vi "Create_Dataset(In3d_Out3D).vi"(4 "Read GTs?":bool, 5 "Input3D_Custom_Dims":T1, 6 "PreProcessing_Options":T2={"Image Type"=4, "Normalization Type"=enum."Standardize(DS_Stats)", "Interpolation Type"=1} {"Interpolation Type" items=["Zero Order", "Bi-Linear", "Quadratic", "Cubic Spline"]; "Image Type" items=["Grayscale (U8)", "Grayscale (I16)", "Grayscale (SGL)", "Complex (CSG)", "RGB (U32)", "HSL (U32)", "RGB (U64)", "Grayscale (U16)"]}, 7 "Dataset_Stats":T5 {"vars"."R" format="%#_3g"; "vars"."G" format="%#_3g"; "vars"."B" format="%#_3g"; "means"."R" format="%#_3g"; "means"."G" format="%#_3g"; "means"."B" format="%#_3g"}, 8 "error in (no error)":errorcluster, 9 "Good Unique Labels":string[](array[string]), 10 "GT Folder Path":path, 11 "Image File Paths":path[](array[path])) -> (0 "error out":errorcluster, 3 "Dataset(In3D_Out3D)":T7)   [LabVIEW 2020]
uses:
  <vilib>/Ngene/Deep Learning Toolkit/Toolkit/NN_Data/API/DataSet/DataSet_Types/NN_DataSet(In3D_Out3D).ctl
  <vilib>/Ngene/Deep Learning Toolkit/Toolkit/NN_Data/API/NN_Dims(C,H,W).ctl
  <vilib>/Ngene/Deep Learning Toolkit/Toolkit/NN_Data/Controls/DataRef_Types/4D/NN_Data_ref(4D_SGL).ctl
  PatchCore_AddOn/API/Controls/NNPC_DS_Stats.ctl
  PatchCore_AddOn/API/Controls/Image_Stats_RGB.ctl
  Controls/ImRead_PreProcessing_Options.ctl
  PatchCore_AddOn/Low_Level/Controls/Normalization_Type.ctl
  <vilib>/Ngene/Deep Learning Toolkit/Toolkit/Deep_Learning_Toolkit_by_Ngene.lvlib
  <vilib>/vision/NI_Vision_Development_Module.lvlib
  PatchCore_AddOn/PatchCore_AddOn.lvlib
panel:
  out "Imgs with missing GT":path[](array[path])
  out "Progress":i32
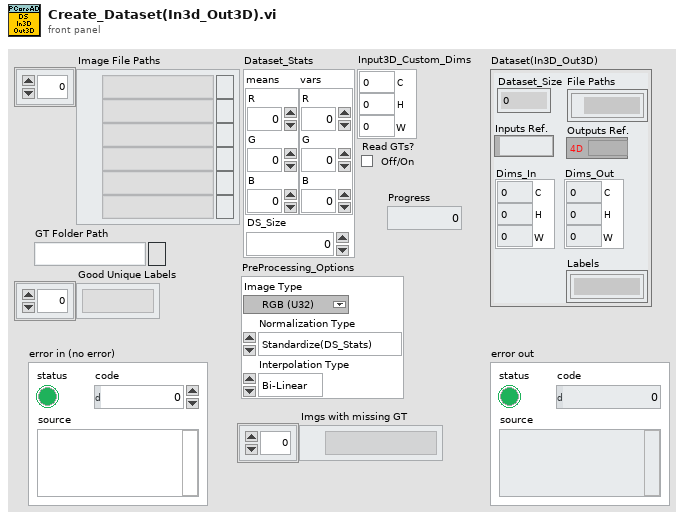
[diagram p1: front panel]
types:
  T1 = typedef "Deep_Learning_Toolkit_by_Ngene.lvlib/NN_Dims(C,H,W).ctl" = cluster{"C":i32, "H":i32, "W":i32}
  T2 = typedef "ImRead_PreProcessing_Options.ctl" = cluster{"Image Type":T3, "Normalization Type":T4, "Interpolation Type":u32}
  T3 = typedef "Image Type" = u32
  T4 = typedef "PatchCore_AddOn.lvlib/Normalization_Type.ctl" = enum16{"Standardize(DS_Stats)", "Standardize(Image_Stats)"}
  T5 = typedef "PatchCore_AddOn.lvlib/NNPC_DS_Stats.ctl" = cluster{"means":T6, "vars":T6, "DS_Size":i32}
  T6 = typedef "PatchCore_AddOn.lvlib/Image_Stats_RGB.ctl" = cluster{"R":sgl, "G":sgl, "B":sgl}
  T7 = typedef "Deep_Learning_Toolkit_by_Ngene.lvlib/NN_DataSet(In3D_Out3D).ctl" = cluster{"Dataset_Size":i32, "Dims_In":T1, "Labels":string[], "File Paths":path[], "Outputs Ref.":T8, "Inputs Ref.":variant, "Dims_Out":T1}
  T8 = typedef "Deep_Learning_Toolkit_by_Ngene.lvlib/NN_Data_ref(4D_SGL).ctl" = refnum<data-value>
  T9 = typedef "IMAQ Image.ctl" = refnum<image>
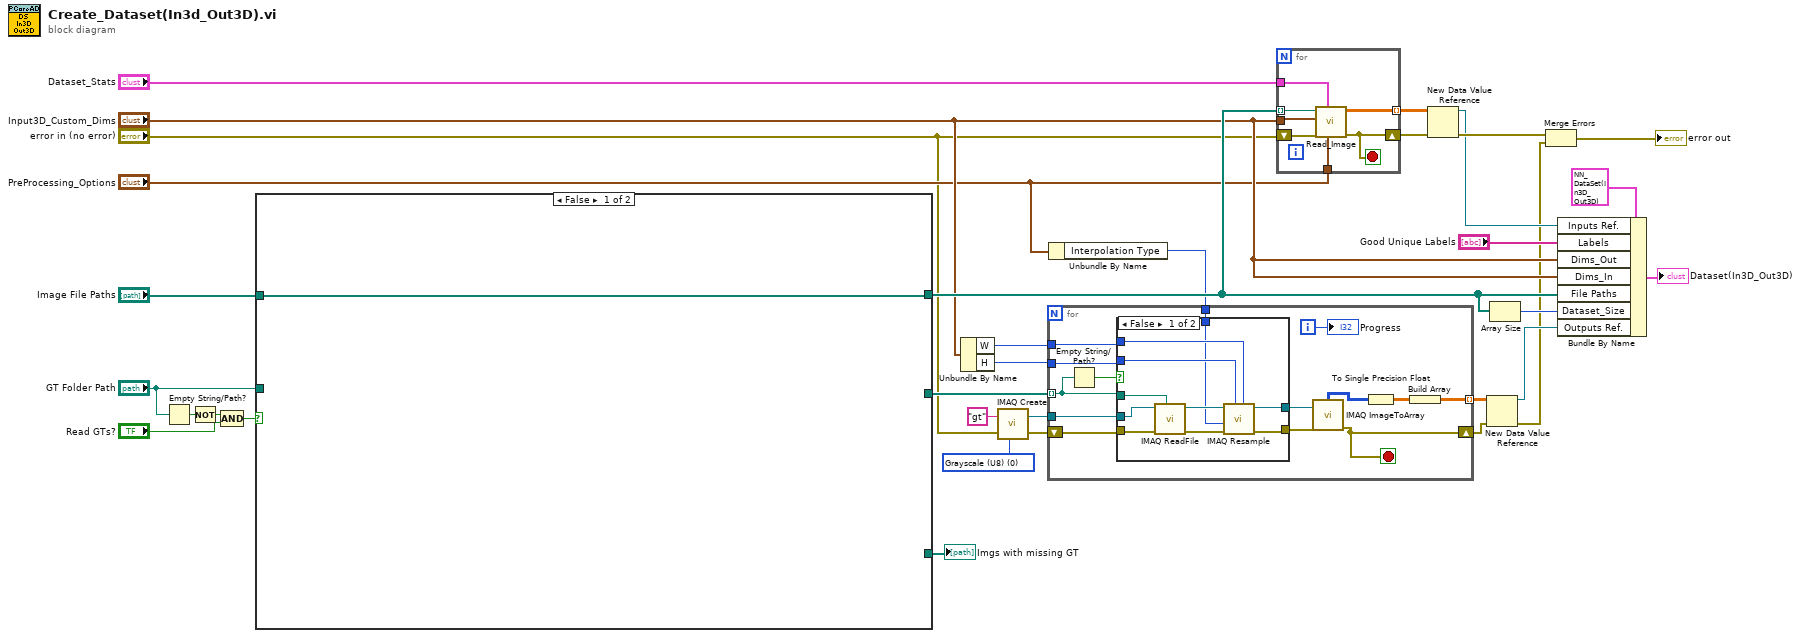
[diagram p0: block diagram]
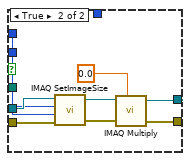
[diagram p2: hidden frame]
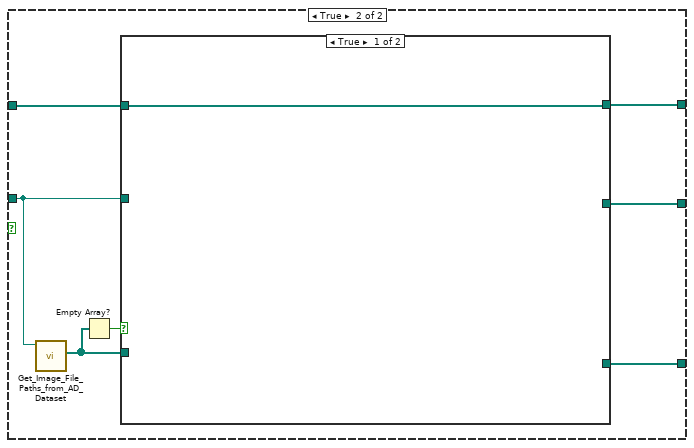
[diagram p3: hidden frame]
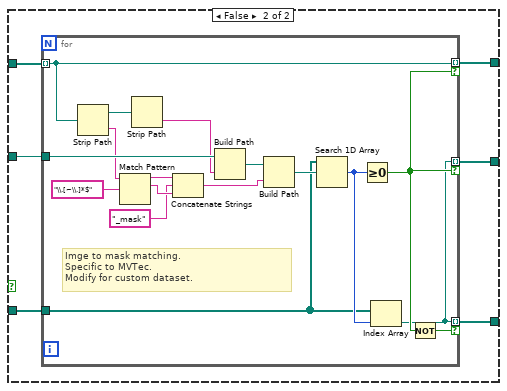
[diagram p4: hidden frame]
diagram:
  w18 = T3 0 items=["Grayscale (U8)", "Grayscale (I16)", "Grayscale (SGL)", "Complex (CSG)", "RGB (U32)", "HSL (U32)", "RGB (U64)", "Grayscale (U16)"] ("Image Type")
  n1 = Empty String/Path?(string/path="GT Folder Path") -> (empty?=w13:bool)
  n2 = Not(x=w13) -> (.not. x?=w12:bool)
  n3 = Compound Arithmetic op=AND(w12, "Read GTs?") -> (w9:bool)
  n4 = case shown="False" w9 {
    tunnel: "GT Folder Path" -> [_ w37]
    tunnel: "Image File Paths" -> [w34 w41]
    tunnel: [_ w40] -> w14
    tunnel: [w34 w39] -> w7
    tunnel: [_ w38] -> w15
    frame False {
    }
    frame True {
      n5 = call "Get_Image_File_Paths_from_AD_Dataset.vi"("Dataset Folder"=w37) -> ("Bad Dataset Files"=w36:path[])  [unwired: 8 in, 2 out]
      n6 = Empty Array?(array=w36) -> (empty?=w35:bool)
      n7 = case shown="True" w35 {
        tunnel: w41 -> [w42 w48]
        tunnel: [_ w47] -> w40
        tunnel: [w42 w46] -> w39
        tunnel: [_ w45] -> w38
        tunnel: w36 -> [_ w44]
        tunnel: w37 -> [_ w43]
        frame True {
        }
        frame False {
          n8 = for {
            tunnel: w44 -> [w52]
            tunnel: w43 -> [w61]
            tunnel: w48 -> [w53] mode=indexing
            tunnel: [w53] -> w46 mode=indexing if=w51
            tunnel: [w49] -> w47 mode=indexing if=w51
            tunnel: [w49] -> w45 mode=indexing if=w50
            # "Imge to mask matching.\nSpecific to MVTec.\nModify for custom dataset."
            n9 = Strip Path(path=w53) -> (stripped path=w60:path, name=w57:string)
            n10 = Match Pattern(string=w57, regular expression="\\.[~\\.]*$") -> (before substring=w64:string, match substring=w65:string)  [unwired: 3 out]
            n11 = Strip Path(path=w60) -> (name=w59:string)  [unwired: 1 out]
            n12 = Concatenate Strings(w64, "_mask" ("string"), w65) -> (w56:string)
            n13 = Build Path(base path=w61, name or relative path=w59) -> (appended path=w58:path)
            n14 = Build Path(base path=w58, name or relative path=w56) -> (appended path=w55:path)
            n15 = Search 1D Array(1D array=w52, element=w55) -> (index of element=w54:i32)  [unwired: 1 in]
            n16 = Greater Or Equal To 0?(x=w54) -> (x >= 0?=w51:bool)
            n17 = Index Array(array=w52, index=w54) -> (element=w49:path)
            n18 = Not(x=w51) -> (.not. x?=w50:bool)
          }
        }
      }
    }
  }
  "Imgs with missing GT" <- w15
  n19 = Unbundle By Name("Input3D_Custom_Dims") -> ("W"=w20:i32, "H"=w19:i32)
  n20 = call "IMAQ Create"("Image Name"="gt", "Image Type"=w18, "error in (no error)"="error in (no error)") -> ("New Image"=w24:T9, "error out"=w22:errorcluster)  [unwired: 2 in]
  n21 = Unbundle By Name("PreProcessing_Options") -> ("Interpolation Type"=w4:u32)
  n22 = for {
    tunnel: w24 -> [w79]
    tunnel: w14 -> [w74] mode=indexing
    tunnel: [w73] -> w17 mode=indexing
    tunnel: w20 -> [w76]
    tunnel: w19 -> [w75]
    tunnel: w4 -> [w67]
    shift-right: [w68] -> w21
    shift-left: w22 -> [w77]
    i -> [w72]
    stop <- w68 stop-if-true
    n23 = Empty String/Path?(string/path=w74) -> (empty?=w78:bool)
    n24 = case shown="False" w78 {
      tunnel: w79 -> [w89 w98]
      tunnel: w77 -> [w88 w97]
      tunnel: [w87 w93] -> w71
      tunnel: [w85 w92] -> w70
      tunnel: w76 -> [w82 w91]
      tunnel: w75 -> [w81 w90]
      tunnel: w74 -> [w83 _]
      tunnel: w67 -> [w80 _]
      frame False {
        n25 = call "IMAQ ReadFile"("File Path"=w83, "error in (no error)"=w88, "Image"=w89) -> ("error out"=w86:errorcluster, "Image Out"=w84:T9)  [unwired: 4 in, 3 out]
        n26 = call "IMAQ Resample"("X Resolution"=w82, "Y Resolution"=w81, "error in (no error)"=w86, "Interpolation Type"=w80, "Image Src"=w84) -> ("error out"=w85:errorcluster, "Image Dst Out"=w87:T9)  [unwired: 5 in]
      }
      frame True {
        n27 = call "IMAQ SetImageSize"("error in (no error)"=w97, "Y Resolution"=w90, "X Resolution"=w91, "Image"=w98) -> ("error out"=w96:errorcluster, "Image Out"=w95:T9)  [unwired: 1 in]
        n28 = call "IMAQ Multiply"("Image Src A"=w95, "Constant"=0.0, "error in (no error)"=w96) -> ("Image Dst Out"=w93:T9, "error out"=w92:errorcluster)  [unwired: 4 in]
      }
    }
    n29 = call "IMAQ ImageToArray"("error in (no error)"=w70, "Image"=w71) -> ("error out"=w68:errorcluster, "Image Pixels (U8)"=w66:u8[][])  [unwired: 2 in, 3 out]
    n30 = To Single Precision Float(number=w66) -> (single precision float=w69:sgl[][])
    n31 = Build Array(w69) -> (w73:sgl[][][])
    "Progress" <- w72
  }
  n32 = for {
    tunnel: [w105] -> w27 mode=indexing
    tunnel: "Dataset_Stats" -> [w100]
    tunnel: w7 -> [w102] mode=indexing
    tunnel: "PreProcessing_Options" -> [w101]
    tunnel: "Input3D_Custom_Dims" -> [w99]
    shift-right: [w103] -> w32
    shift-left: "error in (no error)" -> [w104]
    stop <- w103 stop-if-true
    n33 = call "Read_Image.vi"("PreProcessing_Options"=w101, "Dataset_Stats"=w100, "error in"=w104, "Target_Dims"=w99, "Img Path"=w102) -> ("error out"=w103:errorcluster, "Image Out"=w105:sgl[][][])  [unwired: 4 in, 1 out]
  }
  n34 = New Data Value Reference(data value=w27, error in=w32) -> (data value reference=w28:refnum<data-value>, error out=w33:errorcluster)
  n35 = New Data Value Reference(data value=w17, error in=w21) -> (data value reference=w16:refnum<data-value>, error out=w1:errorcluster)
  n36 = Array Size(array=w7) -> (size(s)=w30:i32)
  n37 = Merge Errors(w33, w1) -> (→"error out":errorcluster)
  n38 = Bundle By Name(cluster=T7 {"Dataset_Size"=0, "Dims_In"={"C"=0, "H"=0, "W"=0}, "Labels"=[], "File Paths"=[], "Outputs Ref."=refnum, "Inputs Ref."=variant, "Dims_Out"={"C"=0, "H"=0, "W"=0}} ("Dataset(In3D_Out3D)"), "Inputs Ref."=w28, "Labels"="Good Unique Labels", "Dims_Out"="Input3D_Custom_Dims", "Dims_In"="Input3D_Custom_Dims", "File Paths"=w7, "Dataset_Size"=w30, "Outputs Ref."=w16) -> (→"Dataset(In3D_Out3D)":T7)
